vi "mätLoop.vi"(0 "SerialNumber beta":string="27601582", 1 "SerialNumber alpha":string="27601609", 4 "Antal mätningar":i32=6, 5 "beta":dbl[][](array[numeric]), 6 "Tidsfönster [s]":string="10", 7 "alpha":dbl[][](array[numeric]), 8 "Mitt av hysteres [V]":string="2.0", 9 "Hysteresprocent [0|50|100]":string="100", 10 "Trigger slope [POS|NEG]":string="POS", 11 "GPIB Frekvensräknare":string="4") -> (2 "standardavvikelse":dbl[][](array[numeric]), 3 "medelvärde":dbl[][](array[numeric]))   [LabVIEW 2020]
uses:
  C:/Users/melwina/Desktop/NyttProjekt/Thorlabs.MotionControl.Controls.dll
  Thorlabs.MotionControl.Controls.dll
  C:/Users/melwina/Desktop/NyttProjekt/ThorLabs.MotionControl.KCube.DCServoCLI.dll
  ThorLabs.MotionControl.KCube.DCServoCLI.dll
  <vilib>/Analysis/NI_AALBase.lvlib
panel:
  in  "KCubeDCServoControl 2":refnum<k24>(container)
  in  "KCubeDCServoControl":refnum<k24>(container)
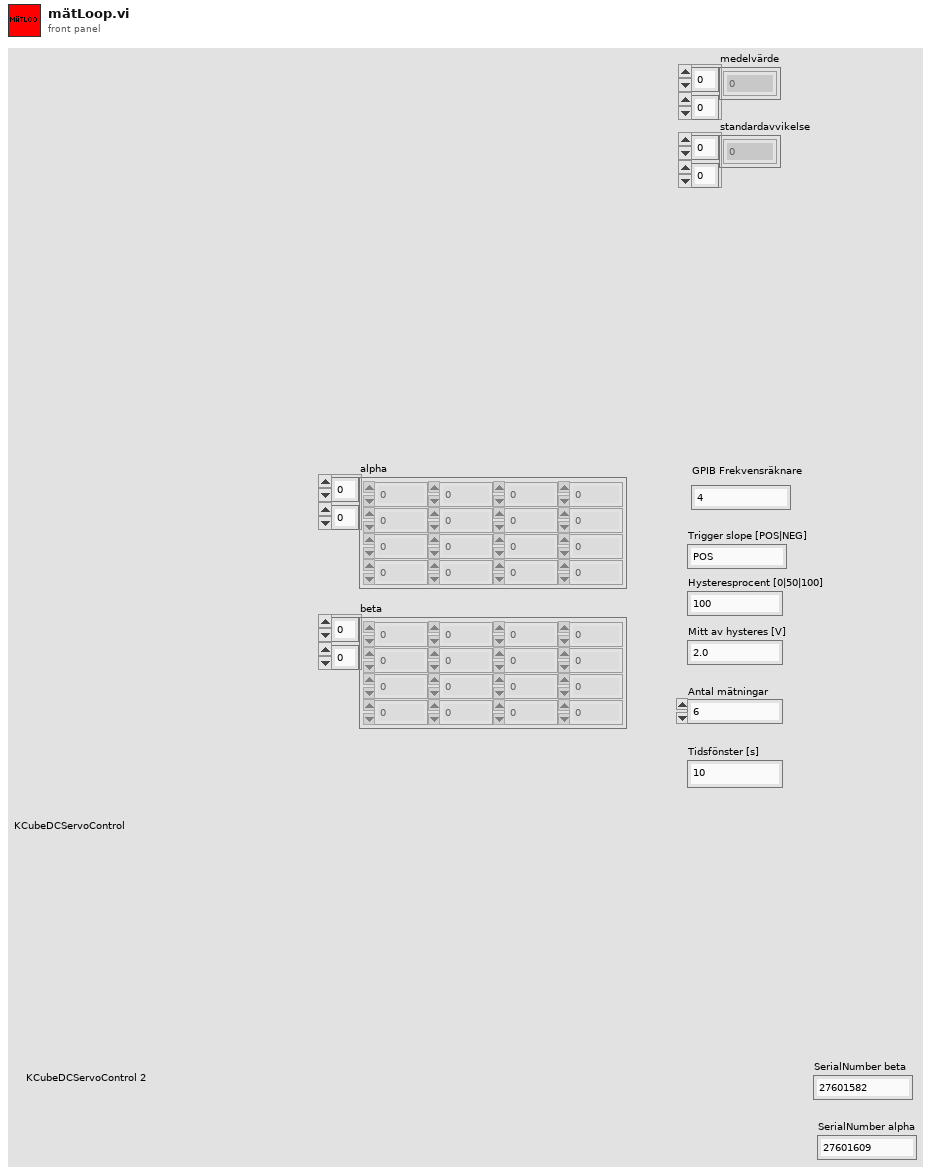
[diagram p1: front panel]
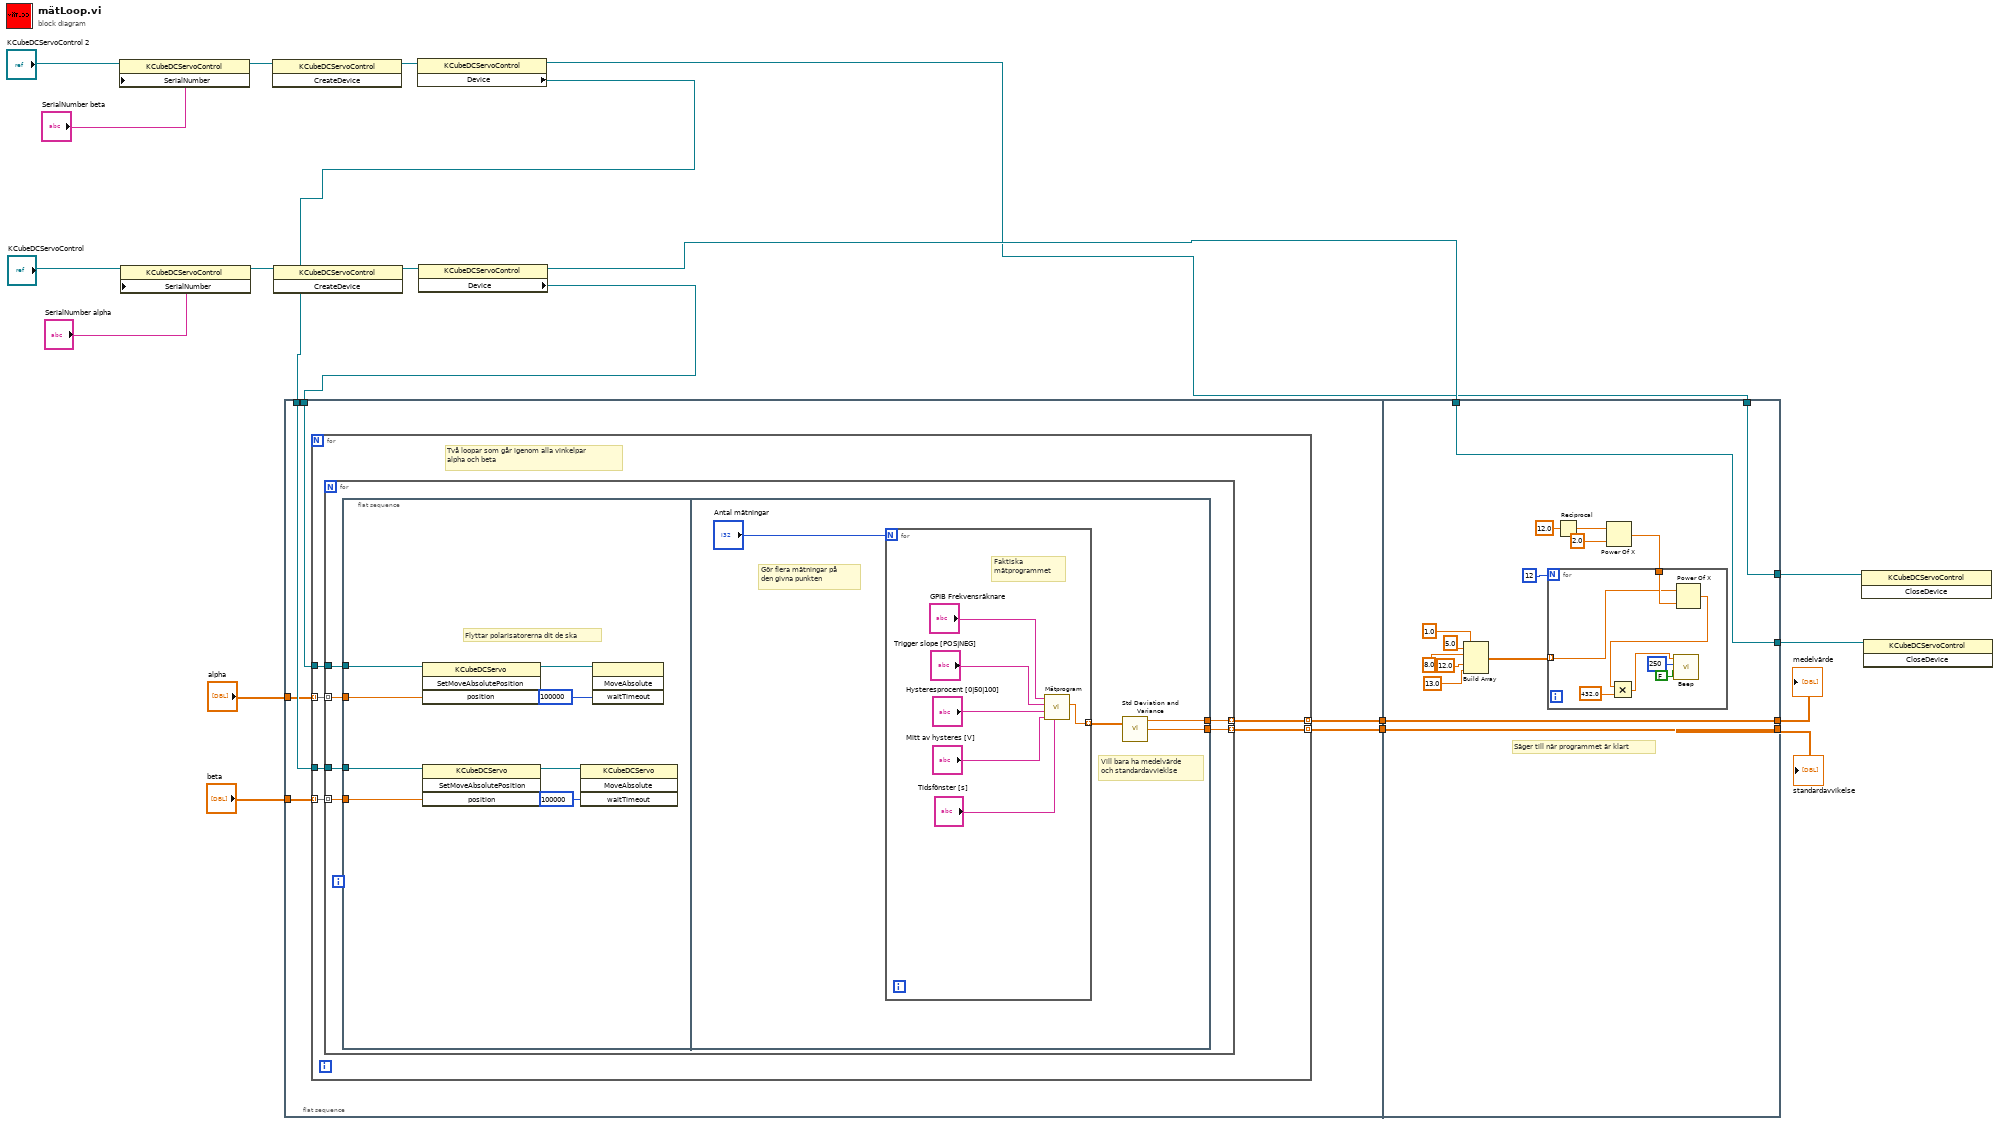
[diagram p0: block diagram]
diagram:
  n1 = property class="KCubeDCServoControl"(reference="KCubeDCServoControl 2", "SerialNumber"="SerialNumber beta") -> (reference out=w13:refnum<k24>)  [unwired: 1 in, 1 out]
  n2 = property class="KCubeDCServoControl"(reference="KCubeDCServoControl", "SerialNumber"="SerialNumber alpha") -> (reference out=w17:refnum<k24>)  [unwired: 1 in, 1 out]
  n3 = invoke class="KCubeDCServoControl" method="CreateDevice"(reference=w13) -> (reference out=w12:refnum<k24>)  [unwired: 2 in, 2 out]
  n4 = invoke class="KCubeDCServoControl" method="CreateDevice"(reference=w17) -> (reference out=w16:refnum<k24>)  [unwired: 2 in, 2 out]
  n5 = flat-sequence {
    tunnel: "beta" -> [w26]
    tunnel: w11 -> [w25]
    tunnel: w10 -> [w24]
    tunnel: [w21] -> w20
    tunnel: "alpha" -> [w23]
    tunnel: [w22] -> w5
    tunnel: [w71] -> w9
    tunnel: [w65] -> w8
    tunnel: w20 -> [w65]
    tunnel: w5 -> [w71]
    tunnel: w3 -> [w58]
    tunnel: [w58] -> w4
    tunnel: w2 -> [w57]
    tunnel: [w57] -> w1
    frame #0 {
      n6 = for {
        tunnel: w26 -> [w32] mode=indexing
        tunnel: w25 -> [w31]
        tunnel: w24 -> [w30]
        tunnel: w23 -> [w29] mode=indexing
        tunnel: [w28] -> w22 mode=indexing
        tunnel: [w27] -> w21 mode=indexing
        # "Två loopar som går igenom alla vinkelpar\nalpha och beta"
        n7 = for {
          tunnel: w32 -> [w38] mode=indexing
          tunnel: [w35] -> w27 mode=indexing
          tunnel: w30 -> [w37]
          tunnel: w31 -> [w36]
          tunnel: [w34] -> w28 mode=indexing
          tunnel: w29 -> [w33] mode=indexing
          n8 = flat-sequence {
            tunnel: w38 -> [w40]
            tunnel: w37 -> [w42]
            tunnel: w36 -> [w41]
            tunnel: w33 -> [w39]
            tunnel: [w49] -> w35
            tunnel: [w48] -> w34
            frame #0 {
              # "Flyttar polarisatorerna dit de ska"
              n9 = invoke class="KCubeDCServo" method="SetMoveAbsolutePosition"(reference=w41, "position"=w39) -> (reference out=w46:refnum<k24>)  [unwired: 2 in, 3 out]
              n10 = invoke class="KCubeDCServo" method="SetMoveAbsolutePosition"(reference=w42, "position"=w40) -> (reference out=w44:refnum<k24>)  [unwired: 2 in, 3 out]
              n11 = invoke class="KCubeDCServo" method="MoveAbsolute"(reference=w44, "waitTimeout"=100000) -> ()  [unwired: 2 in, 4 out]
              n12 = invoke method="MoveAbsolute"(reference=w46, "waitTimeout"=100000) -> ()  [unwired: 2 in, 4 out]
            }
            frame #1 {
              # "Vill bara ha medelvärde \noch standardavvieklse"
              # "Gör flera mätningar på \nden givna punkten"
              n13 = for {
                N: "Antal mätningar" -> [_]
                tunnel: [w51] -> w47 mode=indexing
                # "Faktiska \nmätprogrammet"
                n14 = call "Mätprogram.vi"("Tidsfönster [s]"="Tidsfönster [s]", "Mitt av hysteres [V]"="Mitt av hysteres [V]", "Hysteresprocent [0|50|100]"="Hysteresprocent [0|50|100]", "Trigger slope [POS|NEG]"="Trigger slope [POS|NEG]", "GPIB Frekvensräknare"="GPIB Frekvensräknare") -> ("mätvärde"=w51:dbl)  [unwired: 6 in]
              }
              n15 = call <vilib>:"Std Deviation and Variance.vi"("X"=w47) -> ("mean"=w49:dbl, "standard deviation"=w48:dbl)  [unwired: 1 in, 1 out]
            }
          }
        }
      }
    }
    frame #1 {
      # "Säger till när programmet är klart"
      n16 = Build Array(1.0 ("element"), 5.0 ("element"), 8.0 ("element"), 12.0 ("element"), 13.0 ("element")) -> (w59:dbl[])
      n17 = Reciprocal(x=12.0 ("y")) -> (1/x=w68:dbl)
      n18 = Power Of X(1:2.0, 2:w68) -> (0:w67:dbl)
      n19 = for {
        N: 12 -> [_]
        tunnel: w67 -> [w78]
        tunnel: w59 -> [w75] mode=indexing
        n20 = Power Of X(1:w78, 2:w75) -> (0:w77:dbl)
        n21 = Multiply(x=w77, y=432.0) -> (x*y=w72:dbl)
        n22 = call <vilib>:"Beep.vi"("use system alert? (T)"=FALSE, "duration (msec)"=u32 250, "frequency (Hz)"=w72) -> ()  [unwired: 9 in]
      }
    }
  }
  n23 = property class="KCubeDCServoControl"(reference=w12) -> (reference out=w2:refnum<k24>, "Device"=w10:refnum<k24>)  [unwired: 1 in, 1 out]
  n24 = property class="KCubeDCServoControl"(reference=w16) -> (reference out=w3:refnum<k24>, "Device"=w11:refnum<k24>)  [unwired: 1 in, 1 out]
  n25 = invoke class="KCubeDCServoControl" method="CloseDevice"(reference=w1) -> ()  [unwired: 2 in, 3 out]
  n26 = invoke class="KCubeDCServoControl" method="CloseDevice"(reference=w4) -> ()  [unwired: 2 in, 3 out]
  "medelvärde" <- w8
  "standardavvikelse" <- w9
